vi "Reset Timer.vi"(8 "error in":errorcluster) -> (0 "error out":errorcluster, 1 "New Elapsed Time":dbl, 3 "New Time Stamp":dbl)   [LabVIEW 2023]
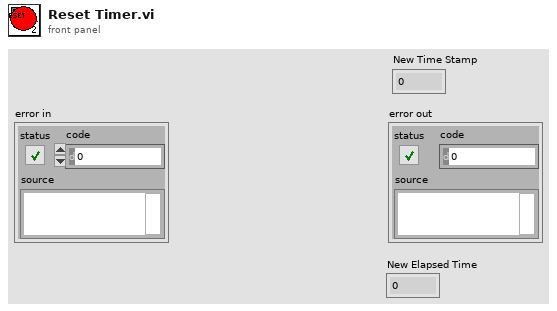
[diagram p1: front panel]
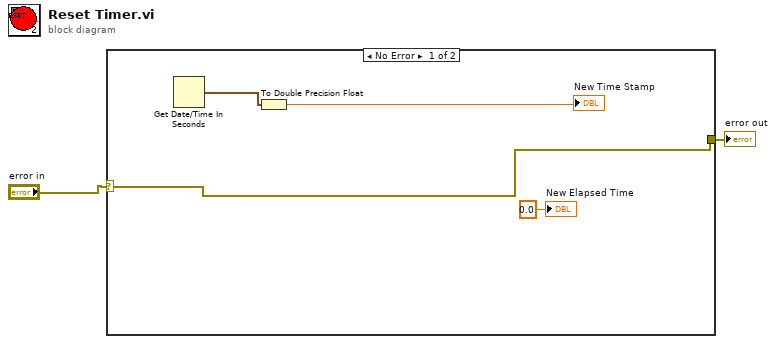
[diagram p0: block diagram]
diagram:
  n1 = case shown="No Error" "error in" {
    selector: "error in" -> [w3 w7]
    tunnel: [w3 w7] -> w1
    frame No Error {
      n2 = Get Date/Time In Seconds() -> (seconds since 1Jan1904=w6:timestamp)
      n3 = To Double Precision Float(number=w6) -> (double precision float=→"New Time Stamp":dbl)
      "New Elapsed Time" <- 0.0 ("New Elapsed Time")
    }
    frame Error {
    }
  }
  "error out" <- w1
